vi "Enque Blocks (SubVI).vi"(0 "Pixels In":u64, 1 "Image Width":u16=3072, 3 "Image Height":u16=3072, 11 "Input Valid?":bool) -> (15 "HT Location":u64[](array[numeric]))   [LabVIEW 2015]
uses:
  Controls (FPGA)/Block Parameters.ctl
  Common/SubVIs (FPGA)/Pixel Bus.ctl
  Controls (FPGA)/Send Blocks.ctl
  <vilib>/rvi/interface/RandomDataEmulation/niFpgaRandomDataHandleErrors.vi
  <vilib>/rvi/Emulation/niFpgaEmulationIsFPGAContextNoSignature.vi
  <vilib>/rvi/Emulation/niFpgaSctlEmulationGetInTimedLoop.vi
  <vilib>/rvi/errors/niFpgaSetErrorForExecOnDevCompSimple.vi
  <vilib>/rvi/eio/common/nirviEmuReportErrorAndStop.vi
  <vilib>/rvi/DataTransferAndStorage/Container/Common/niFpgaContainerGetUniqueNameForEmu.vi
  <vilib>/rvi/FIFO/Fifo_Resource/nirvififoEmulationSetSize.vi
  <vilib>/rvi/FIFO/Fifo_Resource/nirviFifoEmulationQueueMgr.vi
  <instcachedir>/0/nirviFifoEmulationQueueMgr_E5CAEC123FF24DC58D834DCA3CDAA9B5.lvgen/nirviFifoEmulationQueueMgr_E5CAEC123FF24DC58D834DCA3CDAA9B5_001.vi
  <vilib>/Utility/error.llb/Clear Errors.vi
  <vilib>/rvi/FIFO/Fifo_Resource/nirvififoEmulationCreateLock.vi
  <vilib>/rvi/Emulation/niFpgaProcessEmulError.vi
  <vilib>/rvi/FIFO/Fifo_Resource/nirvififoEmulationObtainLock.vi
  <vilib>/rvi/FIFO/Fifo_Resource/nirvififoEmulationReleaseLock.vi
  <vilib>/rvi/occurrence/nirviWaitOnOccurrenceBase.vi
  <vilib>/rvi/errors/nirviReportUnexpectedCaseInternalError.vi
  <vilib>/rvi/errors/nirviReportUnexpectedCaseInternalError (U32).vi
  <vilib>/rvi/FIFO/Fifo_Resource/nirvififoEmulationDetermineInputValidOut.vi
  <vilib>/rvi/DataTransferAndStorage/Container/XNode/niFpgaContainer.xnode
  <vilib>/rvi/interface/RandomDataEmulation/nirviRandomDataFpgaReadWriteTemplate.vi
  <vilib>/rvi/FIFO/Fifo_Resource/nirvififoEmulationRead.vi
  <vilib>/rvi/FIFO/Fifo_Resource/nirvififoEmulationWrite.vi
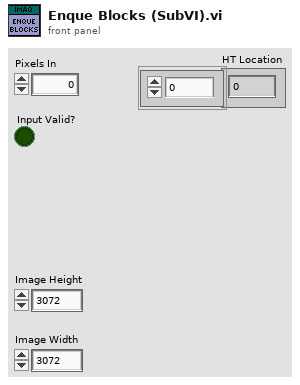
[diagram p1: front panel]
types:
  T1 = typedef "Send Blocks.ctl" = enum8{"Block 1", "2", "3", "4", "5", "6", "7", "8", "9", "10", "11", "12", "13", "14", "15", "16"}
  T2 = typedef "Block Parameters.ctl" = cluster{"Pixels In":u64, "BBox Array":u64[], "Image Height":u16, "Image Width":u16, "Input Valid?":bool, "Pixel Bus":T3}
  T3 = typedef "Pixel Bus.ctl" = cluster{"Pixel Valid":bool, "EOL":bool, "EOF":bool, "X":u16, "Y":u16}
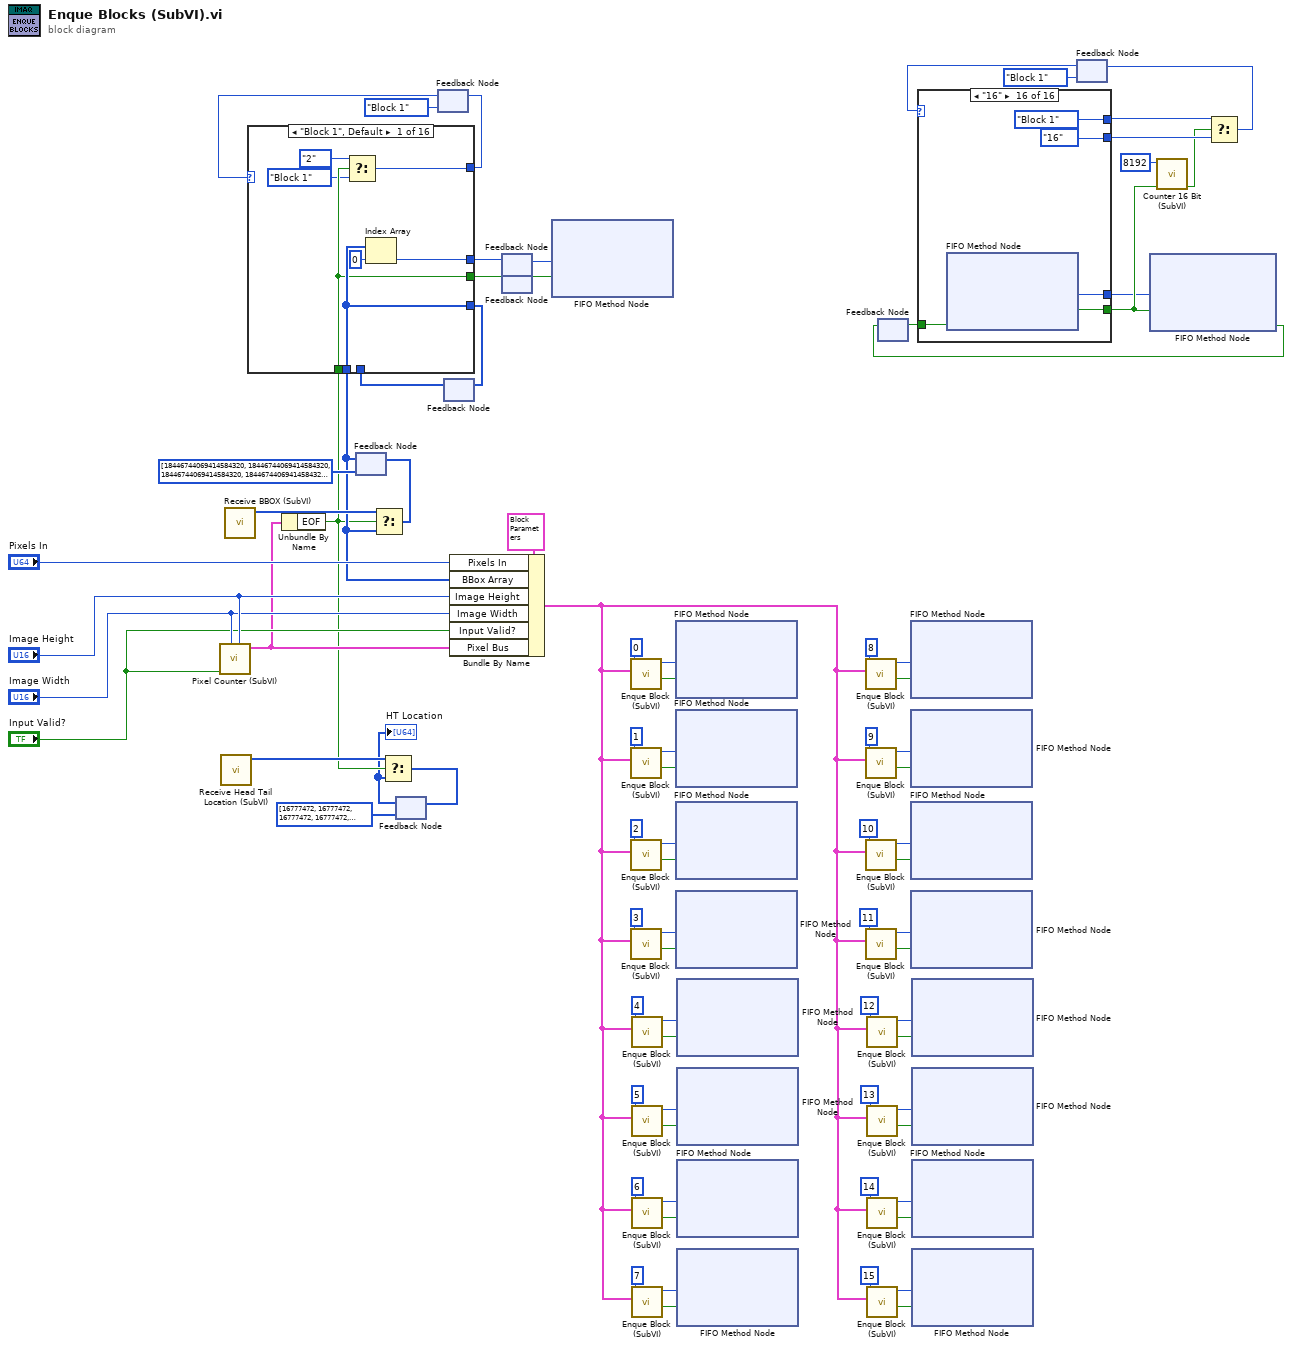
[diagram p0: block diagram]
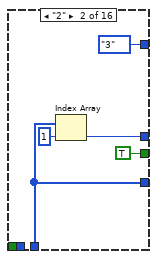
[diagram p2: hidden frame]
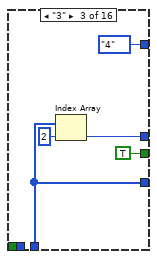
[diagram p3: hidden frame]
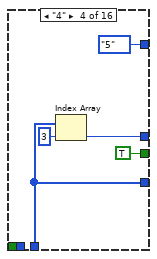
[diagram p4: hidden frame]
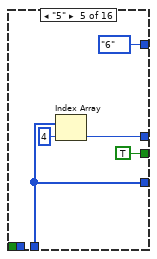
[diagram p5: hidden frame]
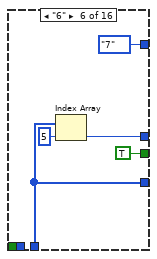
[diagram p6: hidden frame]
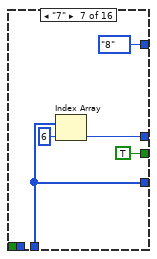
[diagram p7: hidden frame]
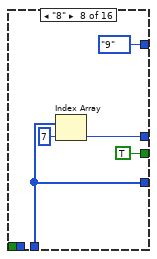
[diagram p8: hidden frame]
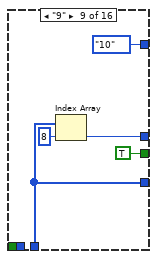
[diagram p9: hidden frame]
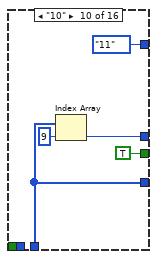
[diagram p10: hidden frame]
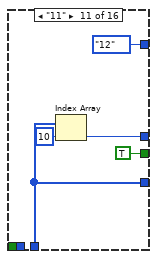
[diagram p11: hidden frame]
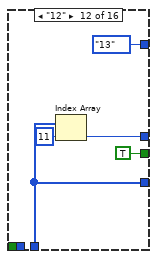
[diagram p12: hidden frame]
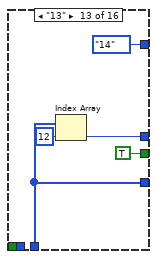
[diagram p13: hidden frame]
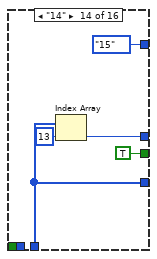
[diagram p14: hidden frame]
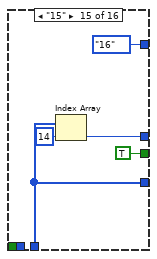
[diagram p15: hidden frame]
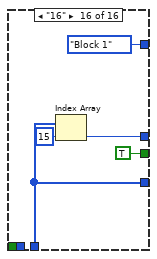
[diagram p16: hidden frame]
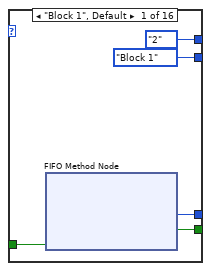
[diagram p17: hidden frame]
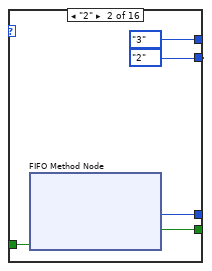
[diagram p18: hidden frame]
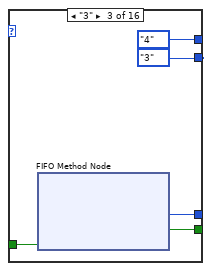
[diagram p19: hidden frame]
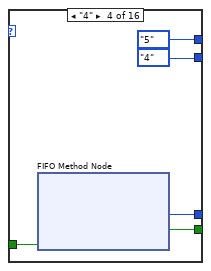
[diagram p20: hidden frame]
diagram:
  n1 = call "Pixel Counter (SubVI).vi"("Image Height"="Image Height", "Image Width"="Image Width", "Pixel Valid"="Input Valid?") -> ("Pixel Bus"=w25:T3)  [unwired: 8 in]
  n2 = call "Receive Head Tail Location (SubVI).vi"() -> ("HT Location"=w5:u64[])  [unwired: 11 in]
  n3 = call "Receive BBOX (SubVI).vi"() -> ("BBox Array"=w17:u64[])  [unwired: 11 in]
  n4 = Unbundle By Name(w25) -> ("EOF"=w4:bool)
  n5 = feedback #1(u64[] [18446744069414584320, 18446744069414584320, 18446744069414584320, 18446744069414584320, 18446744069414584320, 18446744069414584320, 18446744069414584320, 18446744069414584320, 18446744069414584320, 18446744069414584320, 18446744069414584320, 18446744069414584320, 18446744069414584320, 18446744069414584320, 18446744069414584320, 18446744069414584320]) -> (w13:u64[])
  n6 = Select(t=w17, s=w4, f=w13) -> (s? t:f=w24:u64[])
  n7 = feedback-in #1(w24) -> ()
  n8 = feedback #2(u64[] [16777472, 16777472, 16777472, 16777472, 16777472, 16777472, 16777472, 16777472, 16777472, 16777472, 16777472, 16777472, 16777472, 16777472, 16777472, 16777472] ("HT Location")) -> (w1:u64[])
  "HT Location" <- w1
  n9 = Select(t=w5, s=w4, f=w1) -> (s? t:f=w3:u64[])
  n10 = feedback-in #2(w3) -> ()
  n11 = feedback #3(Send_Blocks."Block 1") -> (w15:T1)
  n12 = feedback #4() -> (w11:u64[])  [unwired: 1 in]
  n13 = case shown="\"Block 1\", Default" w15 {
    tunnel: [w91 Send_Blocks."3" ("t") Send_Blocks."4" ("t") Send_Blocks."5" ("t") Send_Blocks."6" ("t") Send_Blocks."7" ("t") Send_Blocks."8" ("t") Send_Blocks."9" ("t") Send_Blocks."10" ("t") Send_Blocks."11" ("t") Send_Blocks."12" ("t") Send_Blocks."13" ("t") Send_Blocks."14" ("t") Send_Blocks."15" ("t") Send_Blocks."16" ("t") Send_Blocks."Block 1"] -> w14
    tunnel: w4 -> [w87 _ _ _ _ _ _ _ _ _ _ _ _ _ _ _]
    tunnel: w13 -> [w89 _ _ _ _ _ _ _ _ _ _ _ _ _ _ _]
    tunnel: [w89 w93 w98 w103 w108 w113 w118 w123 w128 w133 w138 w143 w148 w153 w158 w164] -> w12
    tunnel: [w88 w95 w100 w105 w110 w115 w120 w125 w130 w135 w140 w145 w150 w155 w160 w166] -> w9
    tunnel: [w87 TRUE ("EOF") TRUE ("EOF") TRUE ("EOF") TRUE ("EOF") TRUE ("EOF") TRUE ("EOF") TRUE ("EOF") TRUE ("EOF") TRUE ("EOF") TRUE ("EOF") TRUE ("EOF") TRUE ("EOF") TRUE ("EOF") TRUE ("EOF") TRUE ("EOF")] -> w10
    tunnel: w11 -> [_ w93 w98 w103 w108 w113 w118 w123 w128 w133 w138 w143 w148 w153 w158 w164]
    frame "Block 1", Default {
      n14 = Select(t=Send_Blocks."2", s=w87, f=Send_Blocks."Block 1") -> (s? t:f=w91:T1)
      n15 = Index Array(array=w89, index=0) -> (element=w88:u64)
    }
    frame "2" {
      n16 = Index Array(array=w93, index=1) -> (element=w95:u64)
    }
    frame "3" {
      n17 = Index Array(array=w98, index=2) -> (element=w100:u64)
    }
    frame "4" {
      n18 = Index Array(array=w103, index=3) -> (element=w105:u64)
    }
    frame "5" {
      n19 = Index Array(array=w108, index=4) -> (element=w110:u64)
    }
    frame "6" {
      n20 = Index Array(array=w113, index=5) -> (element=w115:u64)
    }
    frame "7" {
      n21 = Index Array(array=w118, index=6) -> (element=w120:u64)
    }
    frame "8" {
      n22 = Index Array(array=w123, index=7) -> (element=w125:u64)
    }
    frame "9" {
      n23 = Index Array(array=w128, index=8) -> (element=w130:u64)
    }
    frame "10" {
      n24 = Index Array(array=w133, index=9) -> (element=w135:u64)
    }
    frame "11" {
      n25 = Index Array(array=w138, index=10) -> (element=w140:u64)
    }
    frame "12" {
      n26 = Index Array(array=w143, index=11) -> (element=w145:u64)
    }
    frame "13" {
      n27 = Index Array(array=w148, index=12) -> (element=w150:u64)
    }
    frame "14" {
      n28 = Index Array(array=w153, index=13) -> (element=w155:u64)
    }
    frame "15" {
      n29 = Index Array(array=w158, index=14) -> (element=w160:u64)
    }
    frame "16" {
      n30 = Index Array(array=w164, index=15) -> (element=w166:u64)
    }
  }
  n31 = feedback-in #3(w14) -> ()
  n32 = feedback-in #4(w12) -> ()
  n33 = Bundle By Name(cluster=T2 {"Pixels In"=0, "BBox Array"=[0, 0, 0, 0, 0, 0, 0, 0, 0, 0, 0, 0, 0, 0, 0, 0], "Image Height"=3072, "Image Width"=3072, "Input Valid?"=FALSE, "Pixel Bus"={"Pixel Valid"=FALSE, "EOL"=FALSE, "EOF"=FALSE, "X"=0, "Y"=0}}, "Pixels In"="Pixels In", "BBox Array"=w13, "Image Height"="Image Height", "Image Width"="Image Width", "Input Valid?"="Input Valid?", "Pixel Bus"=w25) -> (w34:T2)
  n34 = feedback-in #5(w9) -> ()
  n35 = feedback #5() -> (w8:u64)  [unwired: 1 in]
  n36 = feedback-in #6(w10) -> ()
  n37 = feedback #6() -> (w7:bool)  [unwired: 1 in]
  n38 = xnode ("FIFO Method Node")("Element"=w8, "Input Valid"=w7) -> ()  [unwired: 1 in, 2 out]
  n39 = call "Enque Block (SubVI).vi"("Block Parameters"=w34, "BOX ID"=0) -> ("Pixel Valid?"=w80:bool, "Pixel Data"=w84:u8)  [unwired: 8 in]
  n40 = call "Enque Block (SubVI).vi"("Block Parameters"=w34, "BOX ID"=1) -> ("Pixel Valid?"=w79:bool, "Pixel Data"=w77:u8)  [unwired: 8 in]
  n41 = call "Enque Block (SubVI).vi"("Block Parameters"=w34, "BOX ID"=2) -> ("Pixel Valid?"=w73:bool, "Pixel Data"=w71:u8)  [unwired: 8 in]
  n42 = call "Enque Block (SubVI).vi"("Block Parameters"=w34, "BOX ID"=3) -> ("Pixel Valid?"=w74:bool, "Pixel Data"=w76:u8)  [unwired: 8 in]
  n43 = call "Enque Block (SubVI).vi"("Block Parameters"=w34, "BOX ID"=4) -> ("Pixel Valid?"=w61:bool, "Pixel Data"=w59:u8)  [unwired: 8 in]
  n44 = call "Enque Block (SubVI).vi"("Block Parameters"=w34, "BOX ID"=5) -> ("Pixel Valid?"=w62:bool, "Pixel Data"=w64:u8)  [unwired: 8 in]
  n45 = call "Enque Block (SubVI).vi"("Block Parameters"=w34, "BOX ID"=6) -> ("Pixel Valid?"=w68:bool, "Pixel Data"=w70:u8)  [unwired: 8 in]
  n46 = call "Enque Block (SubVI).vi"("Block Parameters"=w34, "BOX ID"=7) -> ("Pixel Valid?"=w67:bool, "Pixel Data"=w65:u8)  [unwired: 8 in]
  n47 = xnode ("FIFO Method Node")("Element"=w84, "Input Valid"=w80) -> ()  [unwired: 1 in, 2 out]
  n48 = xnode ("FIFO Method Node")("Element"=w77, "Input Valid"=w79) -> ()  [unwired: 1 in, 2 out]
  n49 = xnode ("FIFO Method Node")("Element"=w71, "Input Valid"=w73) -> ()  [unwired: 1 in, 2 out]
  n50 = xnode ("FIFO Method Node")("Element"=w76, "Input Valid"=w74) -> ()  [unwired: 1 in, 2 out]
  n51 = xnode ("FIFO Method Node")("Element"=w59, "Input Valid"=w61) -> ()  [unwired: 1 in, 2 out]
  n52 = xnode ("FIFO Method Node")("Element"=w64, "Input Valid"=w62) -> ()  [unwired: 1 in, 2 out]
  n53 = xnode ("FIFO Method Node")("Element"=w70, "Input Valid"=w68) -> ()  [unwired: 1 in, 2 out]
  n54 = xnode ("FIFO Method Node")("Element"=w65, "Input Valid"=w67) -> ()  [unwired: 1 in, 2 out]
  n55 = call "Enque Block (SubVI).vi"("Block Parameters"=w34, "BOX ID"=8) -> ("Pixel Valid?"=w37:bool, "Pixel Data"=w35:u8)  [unwired: 8 in]
  n56 = call "Enque Block (SubVI).vi"("Block Parameters"=w34, "BOX ID"=9) -> ("Pixel Valid?"=w38:bool, "Pixel Data"=w40:u8)  [unwired: 8 in]
  n57 = call "Enque Block (SubVI).vi"("Block Parameters"=w34, "BOX ID"=10) -> ("Pixel Valid?"=w44:bool, "Pixel Data"=w46:u8)  [unwired: 8 in]
  n58 = call "Enque Block (SubVI).vi"("Block Parameters"=w34, "BOX ID"=11) -> ("Pixel Valid?"=w43:bool, "Pixel Data"=w41:u8)  [unwired: 8 in]
  n59 = call "Enque Block (SubVI).vi"("Block Parameters"=w34, "BOX ID"=12) -> ("Pixel Valid?"=w56:bool, "Pixel Data"=w58:u8)  [unwired: 8 in]
  n60 = call "Enque Block (SubVI).vi"("Block Parameters"=w34, "BOX ID"=13) -> ("Pixel Valid?"=w55:bool, "Pixel Data"=w53:u8)  [unwired: 8 in]
  n61 = call "Enque Block (SubVI).vi"("Block Parameters"=w34, "BOX ID"=14) -> ("Pixel Valid?"=w49:bool, "Pixel Data"=w47:u8)  [unwired: 8 in]
  n62 = call "Enque Block (SubVI).vi"("Block Parameters"=w34, "BOX ID"=15) -> ("Pixel Valid?"=w50:bool, "Pixel Data"=w52:u8)  [unwired: 8 in]
  n63 = feedback #7() -> (w22:bool)  [unwired: 1 in]
  n64 = xnode ("FIFO Method Node")("Element"=w35, "Input Valid"=w37) -> ()  [unwired: 1 in, 2 out]
  n65 = xnode ("FIFO Method Node")("Element"=w40, "Input Valid"=w38) -> ()  [unwired: 1 in, 2 out]
  n66 = xnode ("FIFO Method Node")("Element"=w46, "Input Valid"=w44) -> ()  [unwired: 1 in, 2 out]
  n67 = xnode ("FIFO Method Node")("Element"=w41, "Input Valid"=w43) -> ()  [unwired: 1 in, 2 out]
  n68 = xnode ("FIFO Method Node")("Element"=w58, "Input Valid"=w56) -> ()  [unwired: 1 in, 2 out]
  n69 = xnode ("FIFO Method Node")("Element"=w53, "Input Valid"=w55) -> ()  [unwired: 1 in, 2 out]
  n70 = xnode ("FIFO Method Node")("Element"=w47, "Input Valid"=w49) -> ()  [unwired: 1 in, 2 out]
  n71 = xnode ("FIFO Method Node")("Element"=w52, "Input Valid"=w50) -> ()  [unwired: 1 in, 2 out]
  n72 = feedback #8(Send_Blocks."Block 1") -> (w32:T1)
  n73 = case shown="\"16\"" w32 {
    tunnel: [w171 w176 w181 w186 w191 w196 w201 w206 w211 w216 w221 w226 w231 w236 w241 w246] -> w19
    tunnel: [w170 w175 w180 w185 w190 w195 w200 w205 w210 w215 w220 w225 w230 w235 w240 w245] -> w20
    tunnel: [Send_Blocks."2" ("t") Send_Blocks."3" ("t") Send_Blocks."4" ("t") Send_Blocks."5" ("t") Send_Blocks."6" ("t") Send_Blocks."7" ("t") Send_Blocks."8" ("t") Send_Blocks."9" ("t") Send_Blocks."10" ("t") Send_Blocks."11" ("t") Send_Blocks."12" ("t") Send_Blocks."13" ("t") Send_Blocks."14" ("t") Send_Blocks."15" ("t") Send_Blocks."16" ("t") Send_Blocks."Block 1" ("t")] -> w30
    tunnel: [Send_Blocks."Block 1" Send_Blocks."2" Send_Blocks."3" Send_Blocks."4" Send_Blocks."5" Send_Blocks."6" Send_Blocks."7" Send_Blocks."8" Send_Blocks."9" Send_Blocks."10" Send_Blocks."11" Send_Blocks."12" Send_Blocks."13" Send_Blocks."14" Send_Blocks."15" Send_Blocks."16"] -> w29
    tunnel: w22 -> [w167 w172 w177 w182 w187 w192 w197 w202 w207 w212 w217 w222 w227 w232 w237 w242]
    frame "Block 1", Default {
      n74 = xnode ("FIFO Method Node")("Ready for Output"=w167) -> ("Element"=w171:u8, "Output Valid"=w170:bool)  [unwired: 1 in, 1 out]
    }
    frame "2" {
      n75 = xnode ("FIFO Method Node")("Ready for Output"=w172) -> ("Element"=w176:u8, "Output Valid"=w175:bool)  [unwired: 1 in, 1 out]
    }
    frame "3" {
      n76 = xnode ("FIFO Method Node")("Ready for Output"=w177) -> ("Element"=w181:u8, "Output Valid"=w180:bool)  [unwired: 1 in, 1 out]
    }
    frame "4" {
      n77 = xnode ("FIFO Method Node")("Ready for Output"=w182) -> ("Element"=w186:u8, "Output Valid"=w185:bool)  [unwired: 1 in, 1 out]
    }
    frame "5" {
      n78 = xnode ("FIFO Method Node")("Ready for Output"=w187) -> ("Element"=w191:u8, "Output Valid"=w190:bool)  [unwired: 1 in, 1 out]
    }
    frame "6" {
      n79 = xnode ("FIFO Method Node")("Ready for Output"=w192) -> ("Element"=w196:u8, "Output Valid"=w195:bool)  [unwired: 1 in, 1 out]
    }
    frame "7" {
      n80 = xnode ("FIFO Method Node")("Ready for Output"=w197) -> ("Element"=w201:u8, "Output Valid"=w200:bool)  [unwired: 1 in, 1 out]
    }
    frame "8" {
      n81 = xnode ("FIFO Method Node")("Ready for Output"=w202) -> ("Element"=w206:u8, "Output Valid"=w205:bool)  [unwired: 1 in, 1 out]
    }
    frame "9" {
      n82 = xnode ("FIFO Method Node")("Ready for Output"=w207) -> ("Element"=w211:u8, "Output Valid"=w210:bool)  [unwired: 1 in, 1 out]
    }
    frame "10" {
      n83 = xnode ("FIFO Method Node")("Ready for Output"=w212) -> ("Element"=w216:u8, "Output Valid"=w215:bool)  [unwired: 1 in, 1 out]
    }
    frame "11" {
      n84 = xnode ("FIFO Method Node")("Ready for Output"=w217) -> ("Element"=w221:u8, "Output Valid"=w220:bool)  [unwired: 1 in, 1 out]
    }
    frame "12" {
      n85 = xnode ("FIFO Method Node")("Ready for Output"=w222) -> ("Element"=w226:u8, "Output Valid"=w225:bool)  [unwired: 1 in, 1 out]
    }
    frame "13" {
      n86 = xnode ("FIFO Method Node")("Ready for Output"=w227) -> ("Element"=w231:u8, "Output Valid"=w230:bool)  [unwired: 1 in, 1 out]
    }
    frame "14" {
      n87 = xnode ("FIFO Method Node")("Ready for Output"=w232) -> ("Element"=w236:u8, "Output Valid"=w235:bool)  [unwired: 1 in, 1 out]
    }
    frame "15" {
      n88 = xnode ("FIFO Method Node")("Ready for Output"=w237) -> ("Element"=w241:u8, "Output Valid"=w240:bool)  [unwired: 1 in, 1 out]
    }
    frame "16" {
      n89 = xnode ("FIFO Method Node")("Ready for Output"=w242) -> ("Element"=w246:u8, "Output Valid"=w245:bool)  [unwired: 1 in, 1 out]
    }
  }
  n90 = xnode ("FIFO Method Node")("Element"=w19, "Input Valid"=w20) -> ("Ready for Input"=w21:bool)  [unwired: 1 in, 1 out]
  n91 = feedback-in #7(w21) -> ()
  n92 = call "Counter 16 Bit (SubVI).vi"("Max. Count"=u16 8192, "Enable"=w20) -> ("Count End?"=w23:bool)  [unwired: 11 in, 2 out]
  n93 = Select(t=w30, s=w23, f=w29) -> (s? t:f=w31:T1)
  n94 = feedback-in #8(w31) -> ()
